vi "MidpointGenerator.vi"(2 "Waypoint":dbl, 3 "Array":dbl[][](array[numeric])) -> (0 "Y":dbl, 1 "X":dbl)   [LabVIEW 2012]
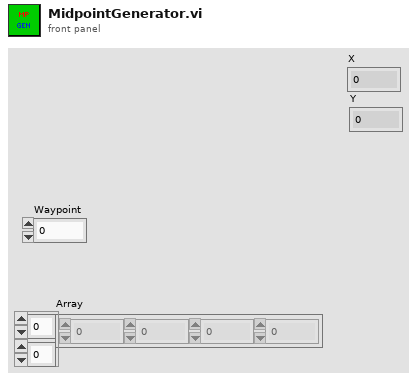
[diagram p1: front panel]
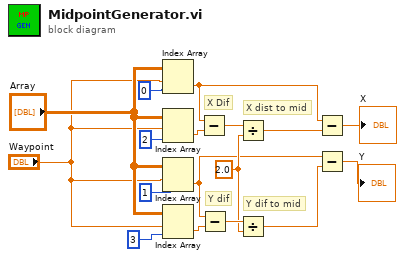
[diagram p0: block diagram]
diagram:
  w12 = 2.0 ("y")
  # "Y dif to mid"
  # "Y dif"
  # "X dist to mid"
  # "X Dif"
  n1 = Index Array(array="Array", index (row)="Waypoint", index (col)=0 ("index")) -> (element=w11:dbl)
  n2 = Index Array(array="Array", index (row)="Waypoint", index (col)=2 ("index")) -> (element=w15:dbl)
  n3 = Index Array(array="Array", index (row)="Waypoint", index (col)=1 ("index")) -> (element=w9:dbl)
  n4 = Index Array(array="Array", index (row)="Waypoint", index (col)=3 ("index")) -> (element=w16:dbl)
  n5 = Subtract(x=w11, y=w15) -> (x-y=w14:dbl)
  n6 = Subtract(x=w9, y=w16) -> (x-y=w13:dbl)
  n7 = Divide(x=w14, y=w12) -> (x/y=w10:dbl)
  n8 = Divide(x=w13, y=w12) -> (x/y=w8:dbl)
  n9 = Subtract(x=w11, y=w10) -> (x-y=→"X":dbl)
  n10 = Subtract(x=w9, y=w8) -> (x-y=→"Y":dbl)
